vi "Create Execution Unit.vi"(8 "error in":errorcluster, 10 "custom device ref":T2=18446744073709551615 format="%.0x", 11 "execution unit factory":refnum<class "Execution Unit Factory.lvclass">) -> (0 "error out":errorcluster, 1 "asynchronous execution units":T1[](array[typedef]) {"ReadWrite Channels" format="%.0x"; "Outgoing Channels" format="%.0x"; "Incoming Channels" format="%.0x"}, 2 "inline execution units":T1[](array[typedef]) {"ReadWrite Channels" format="%.0x"; "Outgoing Channels" format="%.0x"; "Incoming Channels" format="%.0x"}, 3 "execution unit factory out":refnum<class "Execution Unit Factory.lvclass">)   [LabVIEW 2020, in "AIM MIL-STD-1553 Engine.lvlib" / "Implementation.lvlib" / "Execution Unit Factory.lvclass"]
uses:
  Execution Unit Factory.lvclass
  <vilib>/NI VeriStand/Custom Device API/Custom Device Item Ref.ctl
  Interfaces/Controls/Execution Unit Information.ctl
  Interfaces/Execution Unit/Execution Unit.lvclass
  Rx Execution Unit/Rx Execution Unit.lvclass
  C:/dev/git/niveristand-aim-milStd1553-custom-device/Source/Custom Device Support/Engine/Interfaces/Execution Unit/Execution Unit.lvclass
  Tx Execution Unit/Tx Execution Unit.lvclass
  Logging Execution Unit/Logging Execution Unit.lvclass
  Address Based Execution Unit/Address Based Execution Unit.lvclass
  <vilib>/NI VeriStand/Custom Device API/Custom Device API.lvlib
  Interfaces/Interfaces.lvlib
  Execution Unit/Execution Unit.lvclass
  Scripting/AIM MIL-STD-1553 Scripting.lvlib
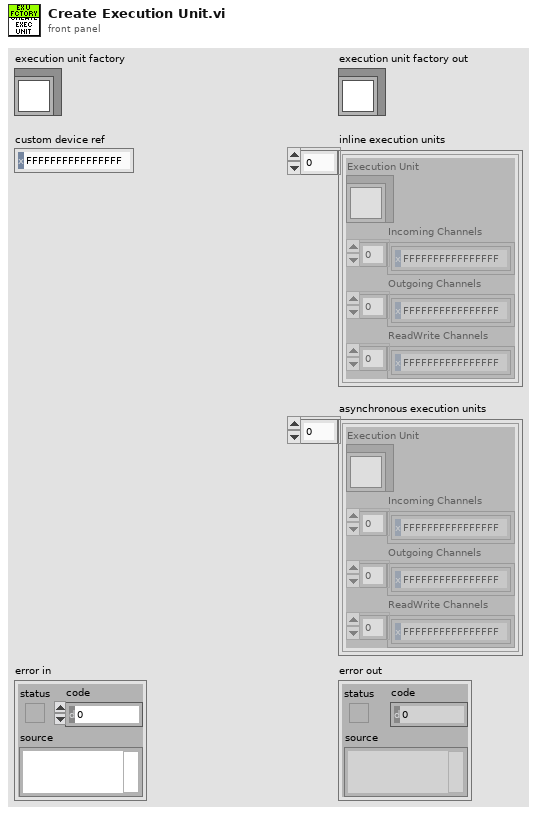
[diagram p1: front panel]
types:
  T1 = typedef "AIM MIL-STD-1553 Engine.lvlib/Interfaces.lvlib/Execution Unit Information.ctl" = cluster{"Execution Unit":refnum<class "Execution Unit.lvclass">, "Incoming Channels":T2[], "Outgoing Channels":T2[], "ReadWrite Channels":T2[]}
  T2 = typedef "Custom Device API.lvlib/Custom Device Item Ref.ctl" = u64
  T3 = typedef "Custom Device API.lvlib/Custom Device Item Info.ctl" = cluster{"Name":string, "Is Channel":bool, "GUID":string, "Is Waveform":bool}
  T4 = typedef "BIU Configuration.ctl" = cluster{"HW channel":u16, "terminal addresses":T5[], "terminal names":string[], "acyclic frame names":string[], "major frames":T6[], "minor frames":T7[], "messages":T8[]}
  T5 = typedef "Address.ctl" = u16
  T6 = typedef "Major Frame Definition.ctl" = cluster{"name":string, "minor frames":string[]}
  T7 = typedef "Minor Frame Definition.ctl" = cluster{"name":string, "messages":string[]}
  T8 = typedef "Message Definition.ctl" = cluster{"name":string, "message type":T9, "endpoint Tx":T10, "endpoint Rx":T10, "create timestamp channel":bool, "mode code":u16, "number of words":u16, "parameters":cluster{"name":string, "default value":dbl, "unit":string, "parameter definition":T11}[]}
  T9 = typedef "Message Type.ctl" = string
  T10 = typedef "Terminal Endpoint.ctl" = cluster{"terminal address":T5, "subaddress":T5}
  T11 = typedef "Parameter Definition.ctl" = cluster{"start index":i32, "size (bits)":i32, "encoding":enum16{"BNR", "BCD", "Discrete"}, "signed":bool, "multiplier":dbl, "offset":dbl}
  T12 = typedef "AIM MIL-STD-1553 Engine.lvlib/Implementation.lvlib/Address Based Execution Unit.lvclass/1553 Address Based Handles.ctl" = cluster{"start stop handles":T13[], "acyclic frame trigger handles":T14[]}
  T13 = typedef "AIM MIL-STD-1553 Engine.lvlib/Implementation.lvlib/Address Based Execution Unit.lvclass/Start Stop Channel Handles.ctl" = cluster{"terminal address":T5, "start handle":T2, "stop handle":T2}
  T14 = typedef "AIM MIL-STD-1553 Engine.lvlib/Implementation.lvlib/Address Based Execution Unit.lvclass/Acyclic Frame Trigger Handle.ctl" = cluster{"name":string, "handle":T2}
  T15 = typedef "AIM MIL-STD-1553 Engine.lvlib/Custom Device.lvlib/Compiled Message.ctl" = cluster{"Message Section Handle":T2, "First Parameter Index":i32, "Parameter Channel Handles":T2[], "Direction":T16, "Parameters":T11[], "Receiving RT Address":u8, "Receiving RT Sub-address":u8, "Transmitting RT Address":u8, "Transmitting RT Sub-address":u8, "Word Count":u8, "Buffer Type":enum16{"unknown", "BC Message Buffer", "RT Message Buffer"}, "Buffer ID":u16, "Terminal Type":enum16{"Bus Controller", "Remote Terminal"}}
  T16 = typedef "Direction.ctl" = enum16{"Rx", "Tx"}
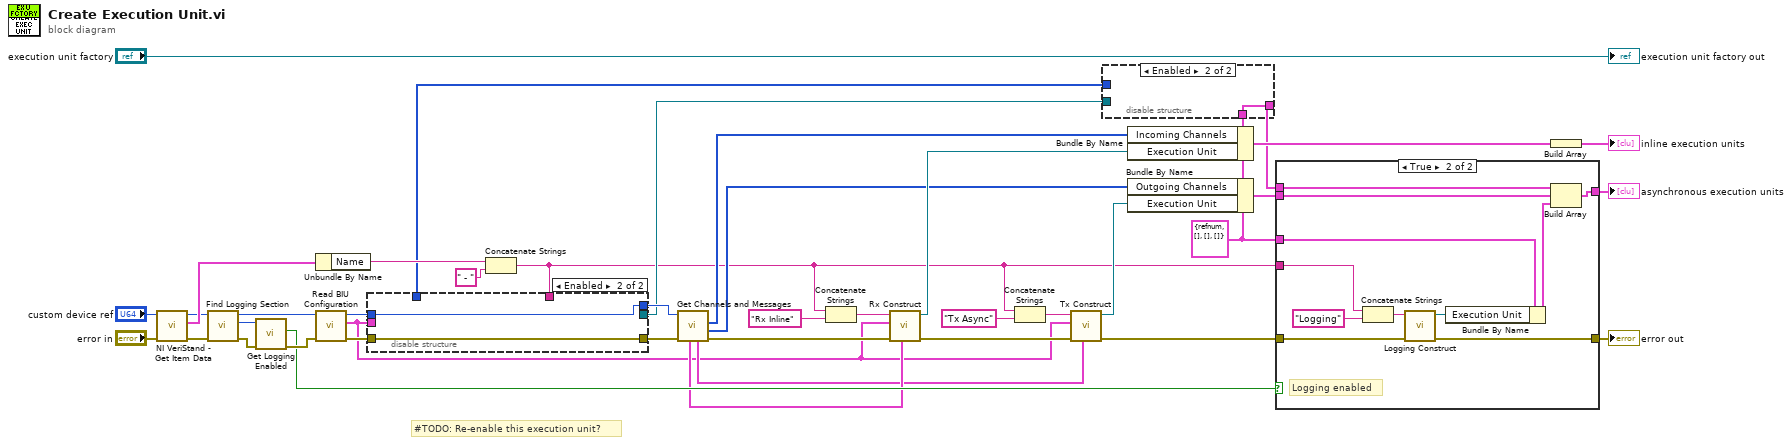
[diagram p0: block diagram]
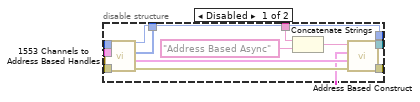
[diagram p2: hidden frame]
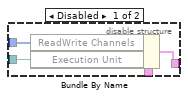
[diagram p3: hidden frame]
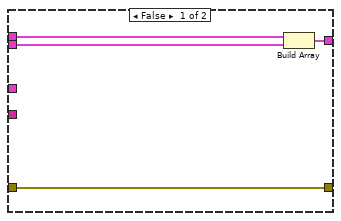
[diagram p4: hidden frame]
diagram:
  w4 = T1 {"Execution Unit"=refnum, "Incoming Channels"=[], "Outgoing Channels"=[], "ReadWrite Channels"=[]} ("Execution Unit Information")
  # "#TODO: Re-enable this execution unit?"
  n1 = call <vilib>:"NI VeriStand - Get Item Data.vi"("error in (no error)"="error in", "Item Ref in"="custom device ref") -> ("error out"=w10:errorcluster, "Item Info"=w25:T3, "Item Ref out"=w8:T2)  [unwired: 6 in, 1 out]
  n2 = call "Find Logging Section.vi"("error in"=w10, "custom device"=w8) -> ("error out"=w9:errorcluster, "logging section"=w11:T2, "custom device out"=w7:T2)  [unwired: 7 in]
  n3 = call "Get Logging Enabled.vi"("error in"=w9, "logging section"=w11) -> ("error out"=w6:errorcluster, "logging enabled"=w5:bool)  [unwired: 7 in, 1 out]
  n4 = Unbundle By Name(w25) -> ("Name"=w24:string)
  n5 = call "Read BIU Configuration.vi"("error in"=w6, "custom device"=w7) -> ("error out"=w32:errorcluster, "biu configuration"=w1:T4, "custom device out"=w33:T2)  [unwired: 7 in]
  n6 = Concatenate Strings(w24, " - " ("string")) -> (w15:string)
  n7 = disable-structure shown="Enabled" {
    disable-tunnel: w33 -> [w53 w54]
    disable-tunnel: w32 -> [w52 w55]
    disable-tunnel: [w50 w55] -> w31
    disable-tunnel: [w49 w54] -> w30
    disable-tunnel: [w48 _] -> w28
    disable-tunnel: [w46 _] -> w17
    disable-tunnel: w15 -> [w43 _]
    disable-tunnel: w1 -> [w42 _]
    frame Disabled {
      n8 = call "1553 Channels to Address Based Handles.vi"("error in"=w52, 10:w42, "custom device ref"=w53) -> ("error out"=w51:errorcluster, "address based channel handles"=w47:T12, "address based channels"=w46:T2[], "custom device ref out"=w49:T2)  [unwired: 5 in]
      n9 = Concatenate Strings(w43, "Address Based Async" ("id")) -> (w44:string)
      n10 = call "Address Based Construct.vi"("error in"=w51, "1553 address based handles"=w47, "biu configuration"=w42, "id"=w44) -> ("error out"=w50:errorcluster, "Address Based Execution Unit Implementation out"=w48:refnum<class "Address Based Execution Unit.lvclass">)  [unwired: 6 in]
    }
    frame Enabled {
    }
  }
  n11 = call "Get Channels and Messages.vi"("error in"=w31, "custom device ref"=w30) -> ("error out"=w35:errorcluster, "outgoing channels"=w16:T2[], "incoming channels"=w36:T2[], "transmitted messages"=w2:T15[], "received messages"=w3:T15[])  [unwired: 4 in, 1 out]
  n12 = Concatenate Strings(w15, "Rx Inline" ("id")) -> (w21:string)
  n13 = call "Rx Construct.vi"("received messages"=w3, "error in"=w35, "biu configuration"=w1, "id"=w21) -> ("error out"=w34:errorcluster, "rx execution unit"=w18:refnum<class "Rx Execution Unit.lvclass">)  [unwired: 6 in]
  n14 = Concatenate Strings(w15, "Tx Async" ("id")) -> (w19:string)
  n15 = call "Tx Construct.vi"("transmitted messages"=w2, "error in"=w34, "biu configuration"=w1, "id"=w19) -> ("error out"=w14:errorcluster, "tx execution unit"=w38:refnum<class "Tx Execution Unit.lvclass">)  [unwired: 6 in]
  n16 = disable-structure shown="Enabled" {
    disable-tunnel: [w59 w60] -> w29
    disable-tunnel: w28 -> [w58 _]
    disable-tunnel: w17 -> [w57 _]
    disable-tunnel: w4 -> [w56 w60]
    frame Disabled {
      n17 = Bundle By Name(cluster=w56, "ReadWrite Channels"=w57, "Execution Unit"=w58) -> (w59:T1)
    }
    frame Enabled {
    }
  }
  n18 = Bundle By Name(cluster=w4, "Incoming Channels"=w36, "Execution Unit"=w18) -> (w40:T1)
  n19 = Bundle By Name(cluster=w4, "Outgoing Channels"=w16, "Execution Unit"=w38) -> (w12:T1)
  n20 = case shown="True" w5 {
    tunnel: [w62 w75] -> w37
    tunnel: w29 -> [w64 w74]
    tunnel: w15 -> [_ w72]
    tunnel: w14 -> [w61 w71]
    tunnel: [w61 w70] -> w13
    tunnel: w12 -> [w63 w68]
    tunnel: w4 -> [_ w65]
    frame False {
      n21 = Build Array(w64, w63) -> (w62:T1[])
    }
    frame True {
      # "Logging enabled"
      n22 = Concatenate Strings(w72, "Logging" ("id")) -> (w69:string)
      n23 = call "Logging Construct.vi"("error in"=w71, "id"=w69) -> ("error out"=w70:errorcluster, "logging execution unit"=w67:refnum<class "Logging Execution Unit.lvclass">)  [unwired: 8 in]
      n24 = Bundle By Name(cluster=w65, "Execution Unit"=w67) -> (w66:T1)
      n25 = Build Array(w74, w68, w66) -> (w75:T1[])
    }
  }
  "error out" <- w13
  "asynchronous execution units" <- w37
  n26 = Build Array(w40) -> (→"inline execution units":T1[])
  "execution unit factory out" <- "execution unit factory"
